vi "FromRepo.vi"(8 "error in":errorcluster, 9 "from repo cluster":T2, 10 "repository in":refnum<class "NISE_CEF_Repository.lvclass">, 11 "node in":refnum<class "NISE_CEF_serializable node.lvclass">) -> (0 "error out":errorcluster, 2 "repository out":refnum<class "NISE_CEF_Repository.lvclass">, 3 "node":T1)   [LabVIEW 2013, in "NISE_CEF_serializable node.lvclass"]
doc: "Grabs information from the Repo and stores it in the nodes."
uses:
  NISE_CEF_serializable node.lvclass
  Repository/NISE_CEF_Repository.lvclass
  Node/FromRepoCluster.ctl
  Node/NodeRef.ctl
  Node/NISE_CEF_Node.lvclass
  hierarchy repo/NISE_CEF_HierarchyRepo.lvclass
  serializable configuration/NISE_CEF_serializable configuration.lvclass
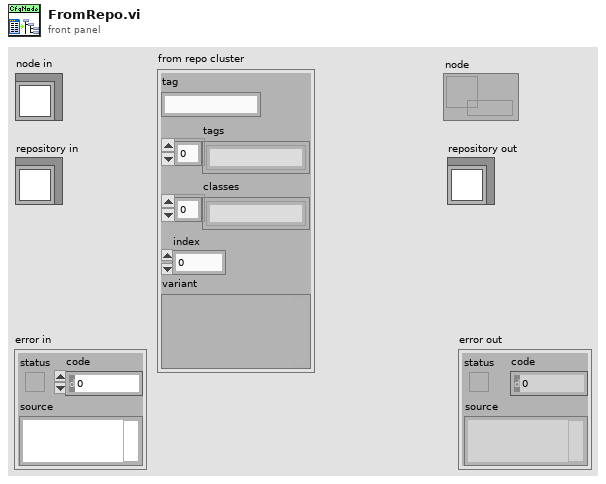
[diagram p1: front panel]
types:
  T1 = typedef "NISE_CEF_Node.lvclass/NodeRef.ctl" = refnum<data-value>
  T2 = typedef "NISE_CEF_Node.lvclass/FromRepoCluster.ctl" = cluster{"tag":string, "tags":string[], "classes":string[], "index":i32, "variant":variant}
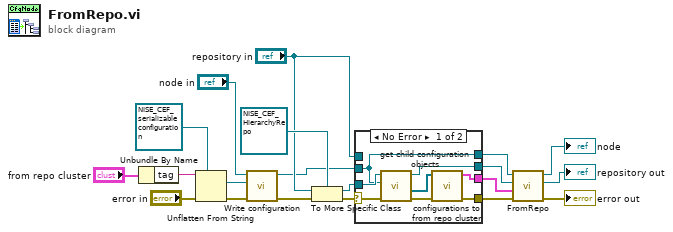
[diagram p0: block diagram]
diagram:
  n1 = Unbundle By Name("from repo cluster") -> ("tag"=w7:string)
  n2 = Unflatten From String(type=refnum<class "NISE_CEF_serializable configuration.lvclass"> refnum ("configuration"), binary string=w7, error in (no error)="error in") -> (value=w1:refnum<class "NISE_CEF_serializable configuration.lvclass">, error out=w4:errorcluster)  [unwired: 2 in, 1 out]
  n3 = call-dynamic "Write configuration.vi"("error in"=w4, "configuration"=w1, "NISE_CEF_serializable node in"="node in") -> ("error out"=w3:errorcluster, "NISE_CEF_serializable node out"=w2:refnum<class "NISE_CEF_serializable node.lvclass">)  [unwired: 7 in]
  n4 = To More Specific Class(target class=refnum<class "NISE_CEF_HierarchyRepo.lvclass"> refnum ("NISE_CEF_HierarchyRepo.lvclass"), reference="repository in", error in=w3) -> (specific class reference=w18:refnum<class "NISE_CEF_HierarchyRepo.lvclass">, error out=w20:errorcluster)
  n5 = case shown="No Error" w20 {
    selector: w20 -> [w26 w30]
    tunnel: "repository in" -> [_ w31]
    tunnel: [w27 w31] -> w15
    tunnel: [w23 w30] -> w17
    tunnel: w2 -> [w25 w29]
    tunnel: [w25 w29] -> w16
    tunnel: w18 -> [w28 _]
    tunnel: [w21 _] -> w10
    frame No Error {
      n6 = call-dynamic "get child configuration objects.vi"("error in"=w26, "serializable node"=w25, "NISE_CEF_HierarchyRepo in"=w28) -> ("error out"=w24:errorcluster, "children"=w22:refnum<class "NISE_CEF_serializable configuration.lvclass">[], "NISE_CEF_HierarchyRepo out"=w27:refnum<class "NISE_CEF_HierarchyRepo.lvclass">)  [unwired: 6 in]
      n7 = call "configurations to from repo cluster.vi"("error in"=w24, "configurations"=w22) -> ("error out"=w23:errorcluster, "from repo cluster"=w21:T2)  [unwired: 8 in]
    }
    frame Error {
    }
  }
  n8 = call-parent "FromRepo.vi"("error in"=w17, "from repo cluster"=w10, "repository in"=w15, "node in"=w16) -> ("error out"=→"error out":errorcluster, "repository out"=→"repository out":refnum<class "NISE_CEF_Repository.lvclass">, "node"=→"node":T1)  [unwired: 5 in]
